vi "Spawn Food.vi"(11 "World in":refnum<class "World.lvclass">) -> (3 "Particle out":refnum<class "Particle.lvclass">)   [LabVIEW 2020, in "Game.lvclass"]
uses:
  Game.lvclass
  Particle.lvclass
  World/World.lvclass
  Particle/Position.ctl
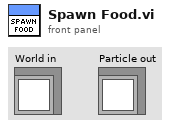
[diagram p1: front panel]
types:
  T1 = typedef "Particle.lvclass/Position.ctl" = cluster{"X":i32, "Y":i32}
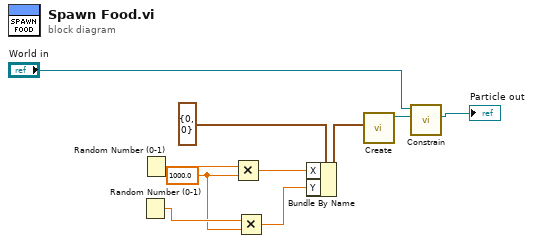
[diagram p0: block diagram]
diagram:
  w4 = 1000.0 ("y")
  n1 = Random Number (0-1)() -> (number: 0 to 1=w5:dbl)
  n2 = Random Number (0-1)() -> (number: 0 to 1=w6:dbl)
  n3 = Multiply(x=w6, y=w4) -> (x*y=w2:dbl)
  n4 = Multiply(x=w5, y=w4) -> (x*y=w1:dbl)
  n5 = Bundle By Name(cluster=T1 {"X"=0, "Y"=0} ("Position"), "X"=w2, "Y"=w1) -> (w3:T1)
  n6 = call "Create.vi"("Position"=w3) -> ("Particle out"=w9:refnum<class "Particle.lvclass">)  [unwired: 10 in]
  n7 = call "Constrain.vi"("Particle.lvclass"=w9, "World in"="World in") -> ("Particle"=→"Particle out":refnum<class "Particle.lvclass">)  [unwired: 8 in, 1 out]
